vi "Read Gain Selection.vi"(8 "error in (no error)":errorcluster, 11 "LINX-ADS1X15 in":refnum<class "LINX-ADS1X15.lvclass">) -> (0 "error out":errorcluster, 2 "Gain Values":T1 items=["+/-6.144V (2/3)"=0, "+/-4.096V (1)"=512, "+/-2.048V (2)"=1024, "+/-1.024V (4)"=1536, "+/-0.512V (8)"=2048, "+/-0.256V (16)"=2560], 3 "LINX-ADS1X15 out":refnum<class "LINX-ADS1X15.lvclass">)   [LabVIEW 2020, in "LINX-ADS1X15.lvclass"]
uses:
  LINX-ADS1X15.lvclass
  Programmable Gain Selection.ctl
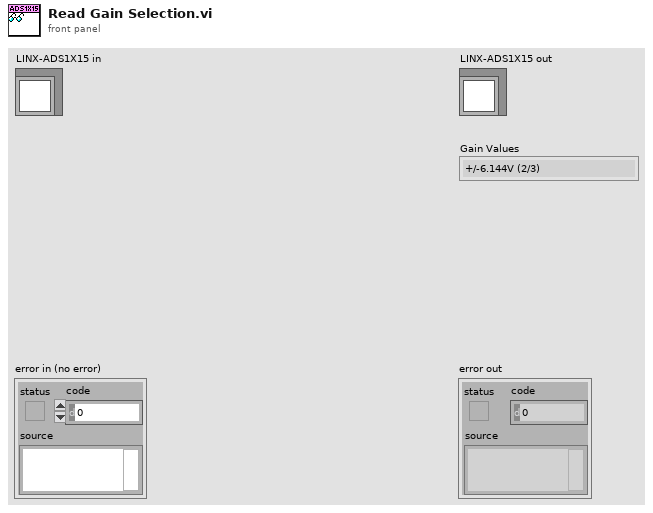
[diagram p1: front panel]
types:
  T1 = typedef "LINX-ADS1X15.lvclass/Programmable Gain Selection.ctl" = u16
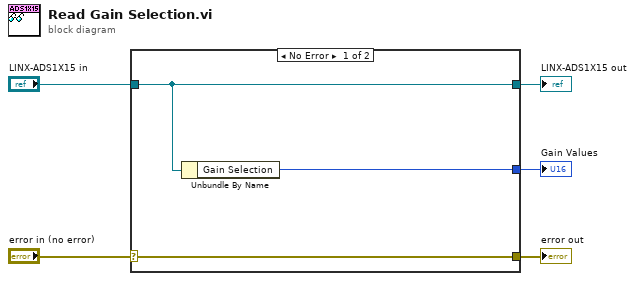
[diagram p0: block diagram]
diagram:
  n1 = case shown="No Error" "error in (no error)" {
    selector: "error in (no error)" -> [w8 w9]
    tunnel: [w8 w9] -> w4
    tunnel: [w7 w10] -> w2
    tunnel: "LINX-ADS1X15 in" -> [w7 w10]
    tunnel: [w6 _] -> w1
    frame No Error {
      n2 = Unbundle By Name(w7) -> ("Gain Selection"=w6:T1)
    }
    frame Error {
    }
  }
  "error out" <- w4
  "LINX-ADS1X15 out" <- w2
  "Gain Values" <- w1
